vi "Destruct Messenger.vi"(8 "error in (no error)":errorcluster, 11 "Queue Messenger Composite in":refnum<class "Simple Tree Queue Messenger.lvclass">) -> (0 "error out":errorcluster, 3 "Queue Messenger Composite out":refnum<class "Simple Tree Queue Messenger.lvclass">)   [LabVIEW 2019, in "Simple Tree Queue Messenger.lvclass"]
uses:
  Simple Tree Queue Messenger.lvclass
  C:/Users/iio/Desktop/NTHU Brain Center/General Library/Ancestor Class/Messenger/Messenger Composite/Messenger Composite.lvclass
  Simple Tree Queue Messenger.lvclass/Simple Tree Queue Messenger.ctl
  Ancestor Class/Messenger/Messenger Composite/Messenger Composite.lvclass/Messenger Composite.ctl
  Ancestor Class/Messenger/Messenger Composite/Public Data/Read Nodes.vi
  Ancestor Class/Messenger/Messenger/Messenger.lvclass
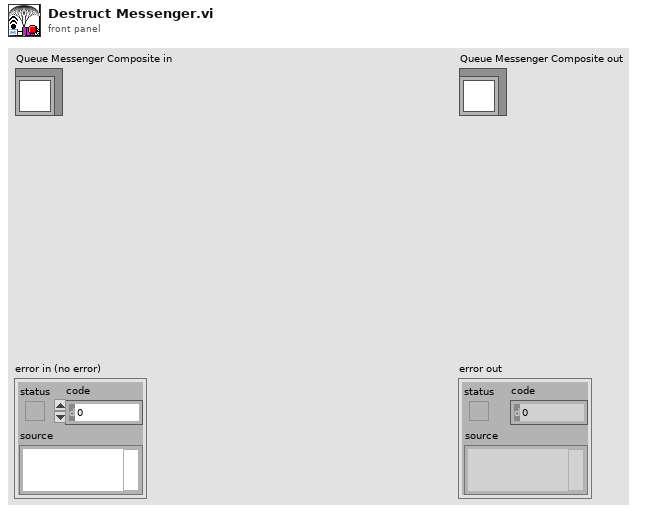
[diagram p1: front panel]
types:
  T1 = typedef "Message Queue.ctl" = refnum<queue>
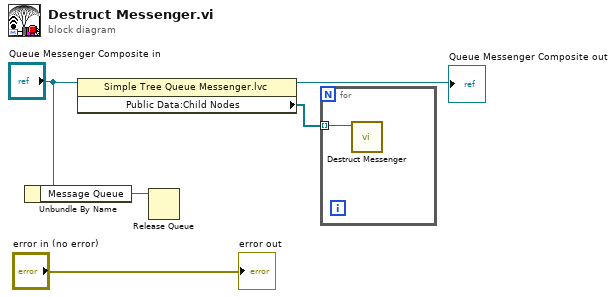
[diagram p0: block diagram]
diagram:
  n1 = Unbundle By Name("Queue Messenger Composite in") -> ("Message Queue"=w4:T1)
  n2 = property class="Simple Tree Queue Messenger.lvc"(reference="Queue Messenger Composite in") -> (reference out=→"Queue Messenger Composite out":refnum<class "Simple Tree Queue Messenger.lvclass">, "Public Data:Child Nodes"=w1:refnum<class "Messenger.lvclass">[])  [unwired: 1 in, 1 out]
  n3 = Release Queue(queue=w4) -> ()  [unwired: 2 in, 3 out]
  n4 = for {
    tunnel: w1 -> [w6] mode=indexing
    n5 = call-dynamic "Destruct Messenger.vi"("Messenger Component in"=w6) -> ()  [unwired: 9 in, 2 out]
  }
  "error out" <- "error in (no error)"
